vi "addDevToTree.vi"(5 "abbrechen":bool, 6 "dev id":i32, 7 "Dev löschen":bool, 8 "error in (no error)":errorcluster, 9 "Elternobjekt-Tag":string, 10 "Tree pics & devs":refnum<vi>, 11 "Device in":refnum<class "Device.lvclass">) -> (0 "error out":errorcluster)   [LabVIEW 2013, in "DataCreation.lvlib"]
uses:
  DataCreation.lvlib
  classes/Datastructure/Device/Device.lvclass
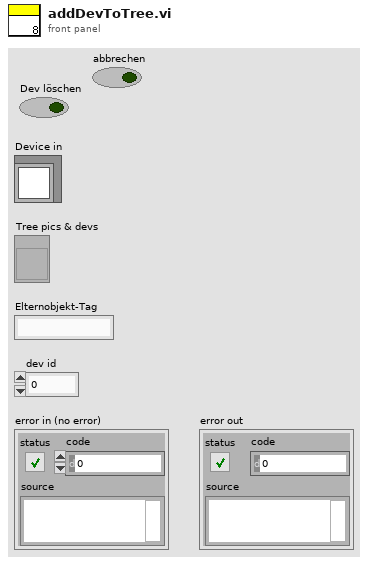
[diagram p1: front panel]
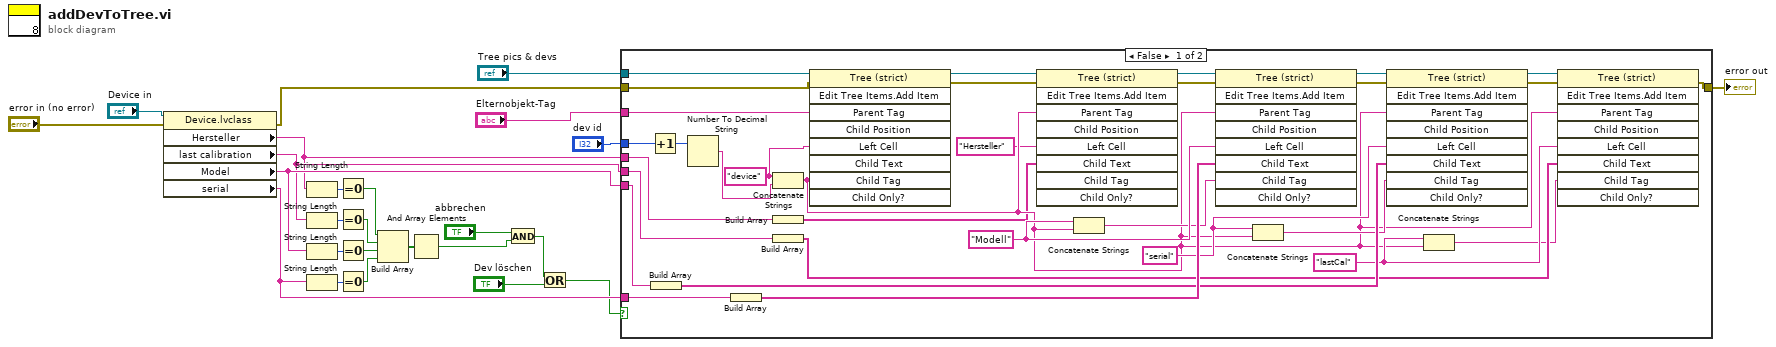
[diagram p0: block diagram]
diagram:
  n1 = property class="Device.lvclass"(reference="Device in", error in="error in (no error)") -> (error out=w22:errorcluster, "Hersteller"=w6:string, "last calibration"=w7:string, "Model"=w8:string, "serial"=w9:string)  [unwired: 1 out]
  n2 = String Length(string=w6) -> (length=w18:i32)
  n3 = String Length(string=w7) -> (length=w17:i32)
  n4 = String Length(string=w8) -> (length=w16:i32)
  n5 = String Length(string=w9) -> (length=w15:i32)
  n6 = Equal To 0?(x=w18) -> (x = 0?=w13:bool)
  n7 = Equal To 0?(x=w17) -> (x = 0?=w14:bool)
  n8 = Equal To 0?(x=w16) -> (x = 0?=w12:bool)
  n9 = Equal To 0?(x=w15) -> (x = 0?=w11:bool)
  n10 = Build Array(w13, w14, w12, w11) -> (w10:bool[])
  n11 = And Array Elements(Boolean array=w10) -> (logical AND=w3:bool)
  n12 = And(x="abbrechen", y=w3) -> (x .and. y?=w2:bool)
  n13 = Or(x=w2, y="Dev löschen") -> (x .or. y?=w1:bool)
  n14 = case shown="False" w1 {
    tunnel: "Elternobjekt-Tag" -> [w55 _]
    tunnel: w9 -> [w30 _]
    tunnel: w8 -> [w50 _]
    tunnel: w7 -> [w49 _]
    tunnel: [w39 w58] -> w19
    tunnel: "Tree pics & devs" -> [w38 _]
    tunnel: w6 -> [w29 _]
    tunnel: w22 -> [w28 w58]
    tunnel: "dev id" -> [w27 _]
    frame False {
      w41 = "lastCal" ("Linker Zellen-String")
      w43 = "serial" ("Linker Zellen-String")
      w45 = "Modell" ("Linker Zellen-String")
      w26 = "device" ("Left Cell String")
      n15 = Increment(x=w27) -> (x+1=w56:i32)
      n16 = Build Array(w50) -> (w47:string[])
      n17 = Number To Decimal String(number=w56) -> (decimal integer string=w57:string)  [unwired: 1 in]
      n18 = Build Array(w30) -> (w48:string[])
      n19 = Concatenate Strings(w26, w57) -> (w33:string)
      n20 = Build Array(w29) -> (w31:string[])
      n21 = Build Array(w49) -> (w46:string[])
      n22 = invoke class="Tree (strict)" method="Edit Tree Items.Add Item"(reference=w38, error in=w28, "Parent Tag"=w55, "Left Cell"=w26, "Child Tag"=w33) -> (reference out=w35:refnum<vi>, error out=w34:errorcluster)  [unwired: 4 in, 7 out]
      n23 = invoke class="Tree (strict)" method="Edit Tree Items.Add Item"(reference=w35, error in=w34, "Parent Tag"=w33, "Left Cell"="Hersteller" ("Left Cell String"), "Child Text"=w31) -> (reference out=w37:refnum<vi>, error out=w36:errorcluster)  [unwired: 4 in, 7 out]
      n24 = Concatenate Strings(w45, w33) -> (w44:string)
      n25 = invoke class="Tree (strict)" method="Edit Tree Items.Add Item"(reference=w37, error in=w36, "Parent Tag"=w33, "Left Cell"=w45, "Child Text"=w48, "Child Tag"=w44) -> (reference out=w54:refnum<vi>, error out=w53:errorcluster)  [unwired: 3 in, 7 out]
      n26 = Concatenate Strings(w43, w33) -> (w42:string)
      n27 = invoke class="Tree (strict)" method="Edit Tree Items.Add Item"(reference=w54, error in=w53, "Parent Tag"=w33, "Left Cell"=w43, "Child Text"=w47, "Child Tag"=w42) -> (reference out=w51:refnum<vi>, error out=w52:errorcluster)  [unwired: 3 in, 7 out]
      n28 = Concatenate Strings(w41, w33) -> (w40:string)
      n29 = invoke class="Tree (strict)" method="Edit Tree Items.Add Item"(reference=w51, error in=w52, "Parent Tag"=w33, "Left Cell"=w41, "Child Text"=w46, "Child Tag"=w40) -> (error out=w39:errorcluster)  [unwired: 3 in, 8 out]
    }
    frame True {
    }
  }
  "error out" <- w19
